vi "FlatToRichhwval_ExportTypeRequest.vi"(5 "OutputClusterType":T1, 11 "InputCluster":T3) -> (3 "OutputCluster":T1)   [LabVIEW 2025, in "Automotive-Vision-OOBService_server.lvlib"]
uses:
  Automotive-Vision-OOBService_server.lvlib
  hwval_ExportTypeRequest_Flat.ctl
  hwval_ExportFileType.ctl
  hwval_ExportTypeRequest.ctl
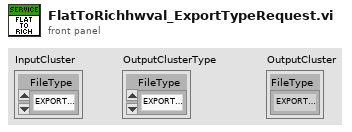
[diagram p1: front panel]
types:
  T1 = typedef "Automotive-Vision-OOBService_server.lvlib/hwval_ExportTypeRequest.ctl" = cluster{"FileType":T2}
  T2 = typedef "Automotive-Vision-OOBService_server.lvlib/hwval_ExportFileType.ctl" = enum32{"EXPORT_PNG", "EXPORT_RAW"}
  T3 = typedef "Automotive-Vision-OOBService_server.lvlib/hwval_ExportTypeRequest_Flat.ctl" = cluster{"FileType":T2}
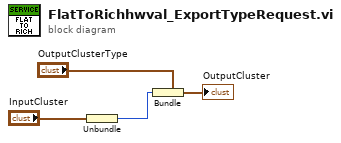
[diagram p0: block diagram]
diagram:
  n1 = Unbundle "Unbundle"("InputCluster") -> ("FileType"=w1:T2)
  n2 = Bundle "Bundle"(cluster="OutputClusterType", "FileType"=w1) -> (→"OutputCluster":T1)
